vi "ConfigureChart.vi"(0 "reference in":refnum<class "LcWebView.lvclass">, 1 "Chart Id":string, 5 "error in (no error)":errorcluster, 6 "Chart Type":T1) -> (14 "reference out":refnum<class "LcWebView.lvclass">, 19 "error out":errorcluster)   [LabVIEW 2018, in "LcWebView.lvclass"]
uses:
  LcWebView.lvclass
  ctrls/ChartType.ctl
  ctrls/ChartConfig.ctl
  fac47259-4e78-44eb-ad12-98a473394377.vi
  <vilib>/JDP Science/JSONtext/Variant to JSON Text.vi
  <vilib>/JDP Science/JSONtext/LVClass Serializer/JSONtext LVClass Serializer.lvclass
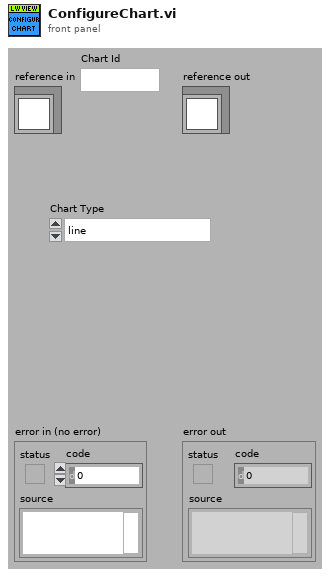
[diagram p1: front panel]
types:
  T1 = typedef "LcWebView.lvclass/ChartType.ctl" = enum16{"line", "bar", "doughnut", "bubble", "scatter", "polarArea", "radar"}
  T2 = typedef "LcWebView.lvclass/ChartContent.ctl" = cluster{"Chart Id":string, "Chart Setup":T3, "Chart HTML":string, "Chart Config":string, "Chart Data":string}
  T3 = typedef "LcWebView.lvclass/ChartSetup.ctl" = cluster{"Chart Id":string, "width":u32, "height":u32}
  T4 = typedef "LcWebView.lvclass/ChartConfig.ctl" = cluster{"type":string, "data":string}
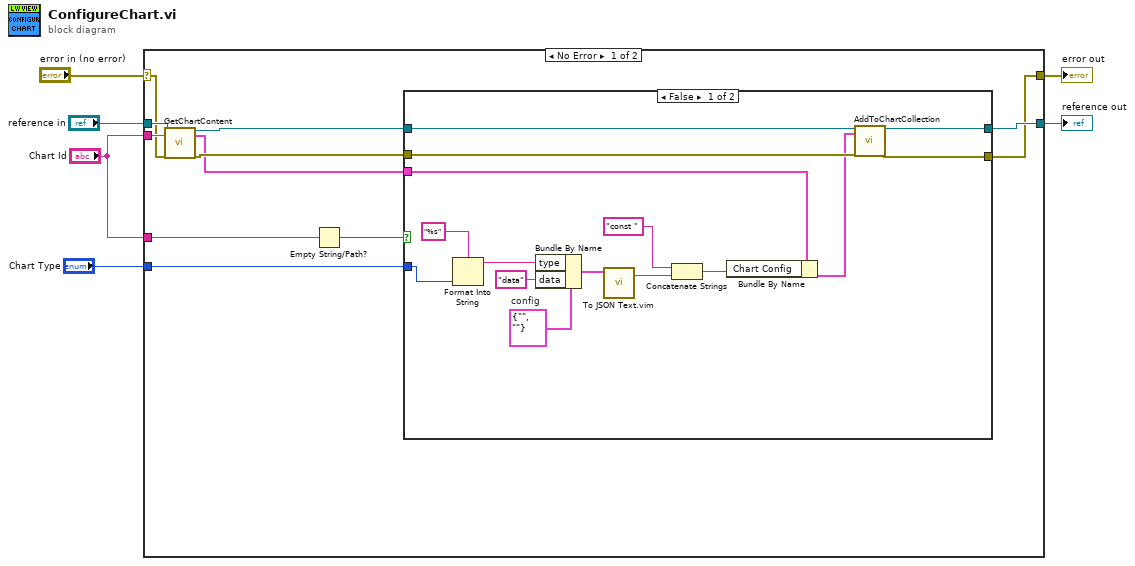
[diagram p0: block diagram]
diagram:
  n1 = case shown="No Error" "error in (no error)" {
    selector: "error in (no error)" -> [w13 w36]
    tunnel: [w11 w36] -> w5
    tunnel: [w14 w35] -> w3
    tunnel: "reference in" -> [w17 w35]
    tunnel: "Chart Id" -> [w16 _]
    tunnel: "Chart Id" -> [w10 _]
    tunnel: "Chart Type" -> [w8 _]
    frame No Error {
      n2 = call-dynamic "GetChartContent.vi"("reference in"=w17, "Chart Id"=w16, "error in (no error)"=w13) -> ("reference out"=w15:refnum<class "LcWebView.lvclass">, "Chart Content"=w7:T2, "error out"=w12:errorcluster)  [unwired: 14 in]
      n3 = Empty String/Path?(string/path=w10) -> (empty?=w9:bool)
      n4 = case shown="False" w9 {
        tunnel: w15 -> [w32 w34]
        tunnel: [w31 w34] -> w14
        tunnel: w12 -> [w30 w33]
        tunnel: [w29 w33] -> w11
        tunnel: w8 -> [w28 _]
        tunnel: w7 -> [w22 _]
        frame False {
          w26 = T4 {"type"="", "data"=""}  # config
          n5 = Format Into String(format string="%s", w28) -> (resulting string=w25:string)  [unwired: 2 in, 1 out]
          n6 = Bundle By Name(cluster=w26, "type"=w25, "data"="data") -> (w23:T4)
          n7 = call "To JSON Text.vim"("Anything"=w23) -> ("<JSON>"=w19:string)  [unwired: 9 in, 1 out]
          n8 = Concatenate Strings("const " ("string"), w19) -> (w18:string)
          n9 = Bundle By Name(cluster=w22, "Chart Config"=w18) -> (w21:T2)
          n10 = call-dynamic "AddToChartCollection.vi"("reference in"=w32, "Chart Content"=w21, "error in (no error)"=w30) -> ("reference out"=w31:refnum<class "LcWebView.lvclass">, "error out"=w29:errorcluster)  [unwired: 15 in]
        }
        frame True {
        }
      }
    }
    frame Error {
    }
  }
  "error out" <- w5
  "reference out" <- w3
